vi "Distance Drive Finished.vi"(11 "Drivetrain Control":T1 {"PID Params"."Y Dist"."output range"."output low" format="%.2f"; "PID Params"."Y Dist"."output range"."output high" format="%.2f"; "PID Params"."Y Dist"."PID gains"."derivative time (Td, min)" format="%.3f"; "PID Params"."Y Dist"."PID gains"."integral time (Ti, min)" format="%.3f"; "PID Params"."Y Dist"."PID gains"."proportional gain (Kc)" format="%.3f"; "PID Params"."X Dist"."output range"."output low" format="%.2f"; "PID Params"."X Dist"."output range"."output high" format="%.2f"; "PID Params"."X Dist"."PID gains"."derivative time (Td, min)" format="%.3f"; "PID Params"."X Dist"."PID gains"."integral time (Ti, min)" format="%.3f"; "PID Params"."X Dist"."PID gains"."proportional gain (Kc)" format="%.3f"}) -> (3 "Finished":bool)   [LabVIEW 2013]
uses:
  Drivetrain Control.ctl
  DT Mode.ctl
  Robot Global Data.vi
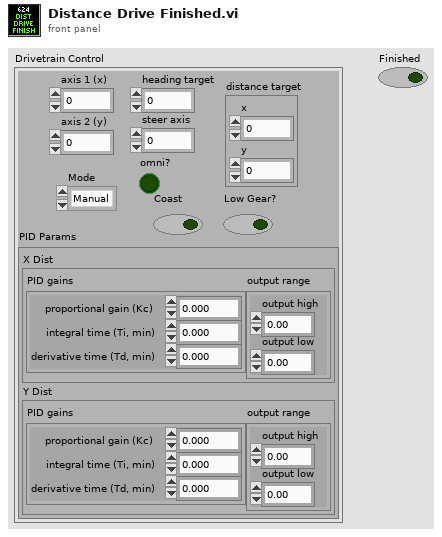
[diagram p1: front panel]
types:
  T1 = typedef "Drivetrain Control.ctl" = cluster{"axis 1 (x)":dbl, "axis 2 (y)":dbl, "Mode":T2, "heading target":dbl, "steer axis":dbl, "omni?":bool, "Low Gear?":bool, "distance target":cluster{"x":dbl, "y":dbl}, "PID Params":cluster{"X Dist":cluster{"PID gains":cluster{"proportional gain (Kc)":dbl, "integral time (Ti, min)":dbl, "derivative time (Td, min)":dbl}, "output range":cluster{"output high":dbl, "output low":dbl}}, "Y Dist":cluster{"PID gains":cluster{"proportional gain (Kc)":dbl, "integral time (Ti, min)":dbl, "derivative time (Td, min)":dbl}, "output range":cluster{"output high":dbl, "output low":dbl}}}, "Coast":bool}
  T2 = typedef "DT Mode.ctl" = enum16{"Manual", "Gyro Steer", "Distance Drive", "Fieldcentric", "Roll Maneuver", "Alt Roll Maneuver"}
  T3 = typedef "Distance Drive Result.ctl" = cluster{"Finished":bool, "distance target":cluster{"x":dbl, "y":dbl}, "Heading Target":dbl, "X Check":bool, "Y Check":bool, "X Dist":dbl, "Y Dist":dbl}
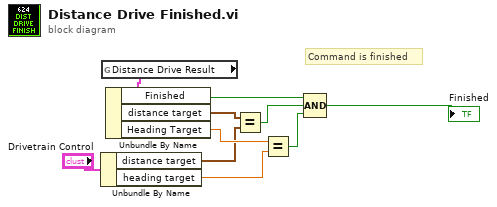
[diagram p0: block diagram]
diagram:
  # "Command is finished"
  n1 = Unbundle By Name("Drivetrain Control") -> ("distance target"=w5:cluster{"x":dbl, "y":dbl}, "heading target"=w7:dbl)
  n2 = global read "Robot Global Data.vi" "Distance Drive Result"() -> (w1:T3)
  n3 = Unbundle By Name(w1) -> ("Finished"=w2:bool, "distance target"=w4:cluster{"x":dbl, "y":dbl}, "Heading Target"=w6:dbl)
  n4 = Equal?(x=w4, y=w5) -> (x = y?=w9:bool)
  n5 = Equal?(x=w6, y=w7) -> (x = y?=w8:bool)
  n6 = Compound Arithmetic op=AND(w2, w9, w8) -> (→"Finished":bool)
